vi "Column Capture Test.vi"() -> (0 "error out":errorcluster)   [LabVIEW 2014, in "SQLite3LV Tests.lvlib"]
uses:
  SQLite3LV Tests.lvlib
  SQLite3LV/Cursor Class/property binding/bind I32.vi
  SQLite3LV/Cursor Class/property binding/column count.vi
  SQLite3LV/Cursor Class/property binding/column I32.vi
  SQLite3LV/SQLite3 Class/sqlite3.lvclass
  SQLite3LV/Cursor Class/cursor.lvclass
panel:
  out "Column Count?":i32
  out "Array":i32[][](array[numeric])
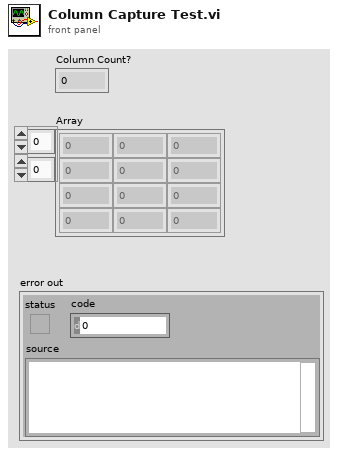
[diagram p1: front panel]
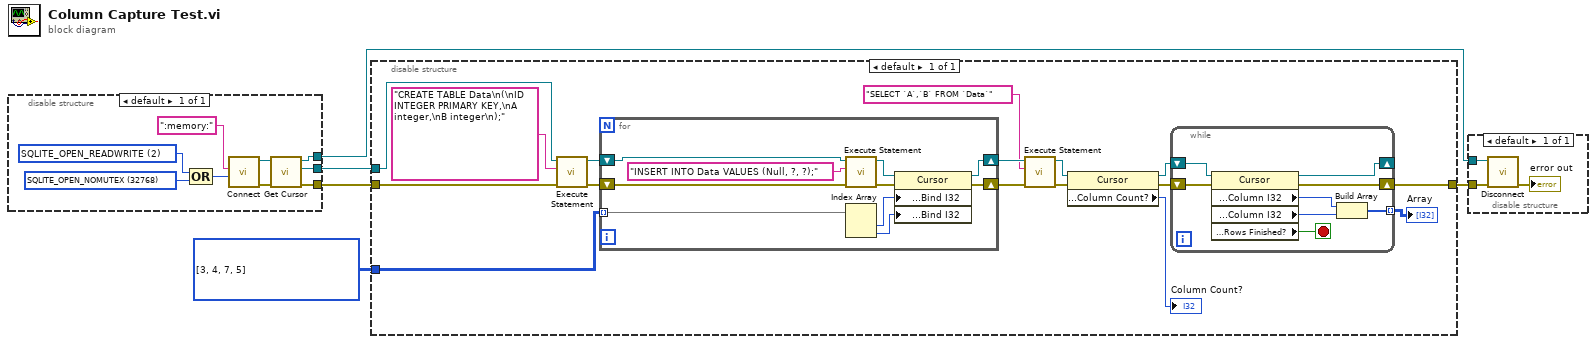
[diagram p0: block diagram]
diagram:
  n1 = disable-structure shown="default" {
    disable-tunnel: [w9] -> w5
    disable-tunnel: [w8] -> w4
    disable-tunnel: [w7] -> w3
    frame Enabled {
      w13 = u32 32768 items=["SQLITE_OPEN_READONLY"=1, "SQLITE_OPEN_READWRITE"=2, "SQLITE_OPEN_CREATE"=4, "SQLITE_OPEN_DELETEONCLOSE"=8, "SQLITE_OPEN_EXCLUSIVE"=16, "SQLITE_OPEN_AUTOPROXY"=32, "SQLITE_OPEN_URI"=64, "SQLITE_OPEN_MEMORY"=128, "SQLITE_OPEN_MAIN_DB"=256, "SQLITE_OPEN_TEMP_DB"=512, "SQLITE_OPEN_TRANSIENT_DB"=1024, "SQLITE_OPEN_MAIN_JOURNAL"=2048, "SQLITE_OPEN_TEMP_JOURNAL"=4096, "SQLITE_OPEN_SUBJOURNAL"=8192, "SQLITE_OPEN_MASTER_JOURNAL"=16384, "SQLITE_OPEN_NOMUTEX"=32768, "SQLITE_OPEN_FULLMUTEX"=65536, "SQLITE_OPEN_SHAREDCACHE"=131072, "SQLITE_OPEN_PRIVATECACHE"=262144, "SQLITE_OPEN_WAL"=524288] ("SQLITE3 Open Flag")
      w14 = u32 2 items=["SQLITE_OPEN_READONLY"=1, "SQLITE_OPEN_READWRITE"=2, "SQLITE_OPEN_CREATE"=4, "SQLITE_OPEN_DELETEONCLOSE"=8, "SQLITE_OPEN_EXCLUSIVE"=16, "SQLITE_OPEN_AUTOPROXY"=32, "SQLITE_OPEN_URI"=64, "SQLITE_OPEN_MEMORY"=128, "SQLITE_OPEN_MAIN_DB"=256, "SQLITE_OPEN_TEMP_DB"=512, "SQLITE_OPEN_TRANSIENT_DB"=1024, "SQLITE_OPEN_MAIN_JOURNAL"=2048, "SQLITE_OPEN_TEMP_JOURNAL"=4096, "SQLITE_OPEN_SUBJOURNAL"=8192, "SQLITE_OPEN_MASTER_JOURNAL"=16384, "SQLITE_OPEN_NOMUTEX"=32768, "SQLITE_OPEN_FULLMUTEX"=65536, "SQLITE_OPEN_SHAREDCACHE"=131072, "SQLITE_OPEN_PRIVATECACHE"=262144, "SQLITE_OPEN_WAL"=524288] ("SQLITE3 Open Flag")
      n2 = Compound Arithmetic op=OR(w14, w13) -> (w11:u32)
      n3 = call "Connect.vi"("SQLITE3 open flags"=w11, "path"=":memory:" ("path_utf8")) -> ("error out"=w6:errorcluster, "SQLite3LV Connection out"=w10:refnum<class "sqlite3.lvclass">)  [unwired: 8 in]
      n4 = call "Get Cursor.vi"("error in (no error)"=w6, "SQLite3LV Connection in"=w10) -> ("error out"=w7:errorcluster, "SQLite3LV Cursor"=w8:refnum<class "cursor.lvclass">, "SQLite3LV Connection out"=w9:refnum<class "sqlite3.lvclass">)  [unwired: 7 in]
    }
  }
  n5 = disable-structure shown="default" {
    disable-tunnel: w4 -> [w24]
    disable-tunnel: w3 -> [w23]
    disable-tunnel: i32[][] [[3, 4], [7, 5]] -> [w22]
    disable-tunnel: [w20] -> w1
    frame Enabled {
      n6 = call "Execute Statement.vi"("error in (no error)"=w23, "SQL statement"="CREATE TABLE Data\n(\nID INTEGER PRIMARY KEY,\nA integer,\nB integer\n);" ("statement"), "SQLite3LV Cursor in"=w24) -> ("error out"=w26:errorcluster, "SQLite3LV Cursor out"=w27:refnum<class "cursor.lvclass">)  [unwired: 7 in]
      n7 = for {
        shift-right: [w43] -> w30
        shift-left: w27 -> [w48]
        shift-right: [w42] -> w29
        shift-left: w26 -> [w46]
        tunnel: w22 -> [w41] mode=indexing
        n8 = call "Execute Statement.vi"("error in (no error)"=w46, "SQL statement"="INSERT INTO Data VALUES (Null, ?, ?);" ("statement"), "SQLite3LV Cursor in"=w48) -> ("error out"=w45:errorcluster, "SQLite3LV Cursor out"=w44:refnum<class "cursor.lvclass">)  [unwired: 7 in]
        n9 = Index Array(array=w41) -> (element #1=w40:i32, element #2=w39:i32)  [unwired: 2 in]
        n10 = property class="Cursor"(reference=w44, error in=w45, "property binding:Bind I32"=w40, "property binding:Bind I32"=w39) -> (reference out=w43:refnum<class "cursor.lvclass">, error out=w42:errorcluster)
      }
      n11 = call "Execute Statement.vi"("error in (no error)"=w29, "SQL statement"="SELECT `A`,`B` FROM `Data`" ("statement"), "SQLite3LV Cursor in"=w30) -> ("error out"=w19:errorcluster, "SQLite3LV Cursor out"=w18:refnum<class "cursor.lvclass">)  [unwired: 7 in]
      n12 = property class="Cursor"(reference=w18, error in=w19) -> (reference out=w17:refnum<class "cursor.lvclass">, error out=w16:errorcluster, "property binding:Column Count?"=→"Column Count?":i32)
      n13 = while {
        shift-right: [w36] -> _
        shift-left: w17 -> [w38]
        shift-right: [w35] -> w20
        shift-left: w16 -> [w37]
        tunnel: [w31] -> w21 mode=indexing
        stop <- w32 stop-if-true
        n14 = property class="Cursor"(reference=w38, error in=w37) -> (reference out=w36:refnum<class "cursor.lvclass">, error out=w35:errorcluster, "property binding:Column I32"=w34:i32, "property binding:Column I32"=w33:i32, "property binding:Rows Finished?"=w32:bool)
        n15 = Build Array(w34, w33) -> (w31:i32[])
      }
      "Array" <- w21
    }
  }
  n16 = disable-structure shown="default" {
    disable-tunnel: w5 -> [w50]
    disable-tunnel: w1 -> [w49]
    frame Enabled {
      n17 = call "Disconnect.vi"("error in (no error)"=w49, "SQLite3LV Connection in"=w50) -> ("error out"=→"error out":errorcluster)  [unwired: 9 in]
    }
  }
